vi "CurImaOneLi.vi"() -> ()   [LabVIEW 2011]
panel:
  in  "Current Image one line":i32[](array[numeric])
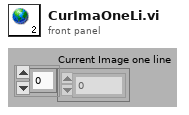
[diagram p1: front panel]
diagram:
